vi "Execute.vi"(0 "reference in":refnum<class "Communication.lvclass">, 2 "Input":string, 5 "error in (no error)":errorcluster) -> (14 "reference out":refnum<class "Communication.lvclass">, 16 "Output":string, 19 "error out":errorcluster)   [LabVIEW 2018, in "Communication.lvclass"]
doc: "This VI executes the command on the input and returns the output.\nThis VI dictates the execution order for executing the command in the input string. (in this case always execute VI)"
uses:
  Communication.lvclass
  Executer_class/Executer.lvclass
  Serializers/Serializer_class/Serializer.lvclass
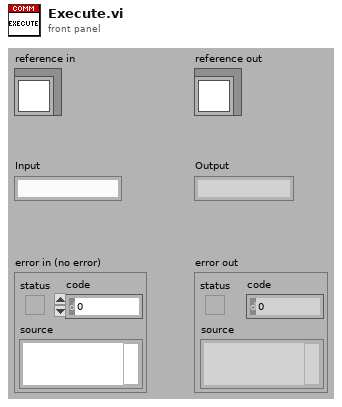
[diagram p1: front panel]
types:
  T1 = typedef "Communication.lvclass/ObjectAttributes.ctl" = cluster{"Executer":refnum<class "Executer.lvclass">, "Serializer":refnum<class "Serializer.lvclass">}
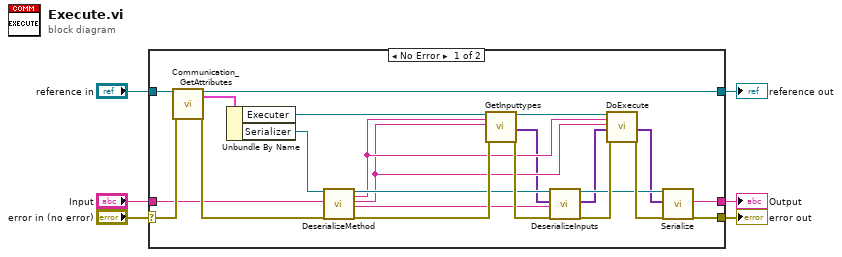
[diagram p0: block diagram]
diagram:
  n1 = case shown="No Error" "error in (no error)" {
    selector: "error in (no error)" -> [w29 w31]
    tunnel: [w22 w31] -> w5
    tunnel: [w26 w30] -> w3
    tunnel: "reference in" -> [w27 w30]
    tunnel: "Input" -> [w20 _]
    tunnel: [w25 _] -> w1
    frame No Error {
      n2 = call "Communication_GetAttributes.vi"("reference in"=w27, "error in (no error)"=w29) -> ("reference out"=w26:refnum<class "Communication.lvclass">, "Data"=w28:T1, "error out"=w24:errorcluster)  [unwired: 14 in, 1 out]
      n3 = Unbundle By Name(w28) -> ("Executer"=w12:refnum<class "Executer.lvclass">, "Serializer"=w21:refnum<class "Serializer.lvclass">)
      n4 = call-dynamic "DeserializeMethod.vi"("object in"=w21, "String"=w20, "error in (no error)"=w24) -> ("object out"=w17:refnum<class "Serializer.lvclass">, "Class"=w15:string, "Method"=w14:string, "Inputsstring"=w9:string, "error out"=w19:errorcluster)  [unwired: 12 in]
      n5 = call-dynamic "GetInputtypes.vi"("reference in"=w12, "Class"=w15, "Method"=w14, "error in (no error)"=w19) -> ("reference out"=w11:refnum<class "Executer.lvclass">, "InputTypes"=w10:variant[], "error out"=w18:errorcluster)  [unwired: 13 in]
      n6 = call-dynamic "DeserializeInputs.vi"("object in"=w17, "Inputtypes"=w10, "InputString"=w9, "error in (no error)"=w18) -> ("object out"=w13:refnum<class "Serializer.lvclass">, "Inputs"=w8:variant[], "error out"=w16:errorcluster)  [unwired: 13 in]
      n7 = call-dynamic "DoExecute.vi"("reference in"=w11, "Class"=w15, "Method"=w14, "Inputs"=w8, "error in (no error)"=w16) -> ("Outputs"=w7:variant[], "error out"=w23:errorcluster)  [unwired: 12 in, 1 out]
      n8 = call-dynamic "Serialize.vi"("object in"=w13, "outputs"=w7, "error in (no error)"=w23) -> ("JSON"=w25:string, "error out"=w22:errorcluster)  [unwired: 14 in, 1 out]
    }
    frame Error {
    }
  }
  "error out" <- w5
  "reference out" <- w3
  "Output" <- w1
